vi "Read Call request.vi"(8 "error in (no error)":errorcluster, 11 "CallRequest (MsgPack) in":refnum<class "CallRequest (MsgPack).lvclass">) -> (0 "error out":errorcluster, 2 "Cluster":T1, 3 "CallRequest (MsgPack) out":refnum<class "CallRequest (MsgPack).lvclass">)   [LabVIEW 2020, in "wamplv.lvlib" / "CallRequest (MsgPack).lvclass"]
uses:
  CallRequest (MsgPack).lvclass
  CallRequest (MsgPack).lvclass/CallRequest (MsgPack).ctl
  MessagePack/MsgPackArray/MsgPackArray.lvclass
  MessagePack/MsgPackMap/MsgPackMap.lvclass
  WAMP Client/API/TypeDefs/WAMP error.ctl
  WAMP Client/WAMP Client.lvclass
  WAMP Client/API/TypeDefs/Combined error.ctl
  WAMP Client/API/TypeDefs/RESULT payload (MsgPack).ctl
  TypeDefs/CALL request (MsgPack).ctl
  wamplv.lvlib
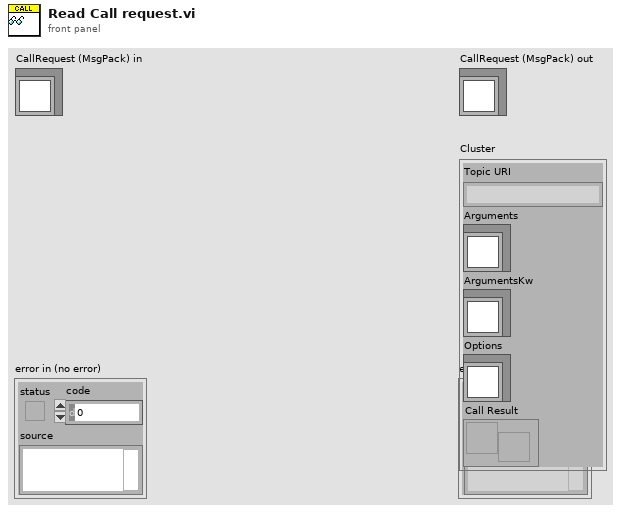
[diagram p1: front panel]
types:
  T1 = typedef "wamplv.lvlib/CALL request (MsgPack).ctl" = cluster{"Topic URI":string, "Arguments":refnum<class "MsgPackArray.lvclass">, "ArgumentsKw":refnum<class "MsgPackMap.lvclass">, "Options":refnum<class "MsgPackMap.lvclass">, "Call Result":refnum<notifier>}
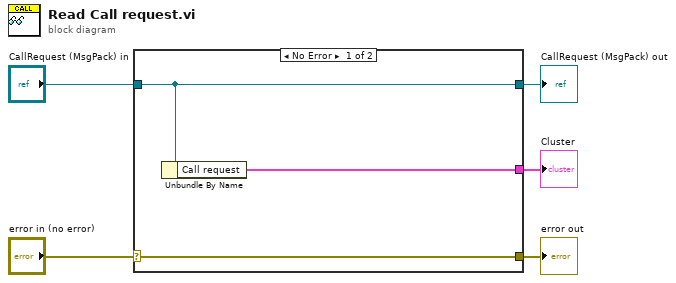
[diagram p0: block diagram]
diagram:
  n1 = case shown="No Error" "error in (no error)" {
    selector: "error in (no error)" -> [w8 w9]
    tunnel: [w8 w9] -> w4
    tunnel: [w7 w10] -> w2
    tunnel: "CallRequest (MsgPack) in" -> [w7 w10]
    tunnel: [w6 _] -> w1
    frame No Error {
      n2 = Unbundle By Name(w7) -> ("Call request"=w6:T1)
    }
    frame Error {
    }
  }
  "error out" <- w4
  "CallRequest (MsgPack) out" <- w2
  "Cluster" <- w1
